vi "Get Error Cluster From DLL Retcode.vi"(8 "error in (no error)":errorcluster, 11 "DLL Return Code":i32 format="%x") -> (0 "error out":errorcluster, 3 "VI Error Code":i32 format="%.0x")   [LabVIEW 2015, in "KEYENCE LJ-X8000A.lvlib"]
doc: "DLLが返すエラーコードをLabVIEWドライバの公開エラーコードに変換する。"
uses:
  KEYENCE LJ-X8000A.lvlib
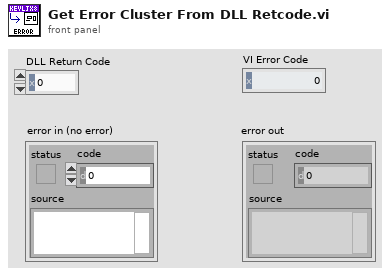
[diagram p1: front panel]
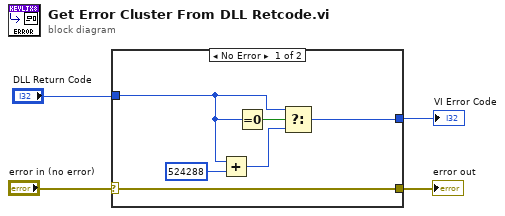
[diagram p0: block diagram]
diagram:
  n1 = case shown="No Error" "error in (no error)" {
    selector: "error in (no error)" -> [w7 w11]
    tunnel: [w7 w11] -> w1
    tunnel: "DLL Return Code" -> [w6 w12]
    tunnel: [w5 w12] -> w2
    frame No Error {
      n2 = Add(x=w6, y=524288) -> (x+y=w8:i32)
      n3 = Equal To 0?(x=w6) -> (x = 0?=w10:bool)
      n4 = Select(t=w6, s=w10, f=w8) -> (s? t:f=w5:i32)
    }
    frame Error {
    }
  }
  "error out" <- w1
  "VI Error Code" <- w2
